vi "Scale sensor data.vi"(7 "Channel type":T1=enum."Flow meter", 11 "RAW Value":dbl) -> (2 "Type name":string, 3 "Scaled value":dbl)   [LabVIEW 2015]
uses:
  Channel type.ctl
  <vilib>/ptbypt/NI_PtbyPt.lvlib
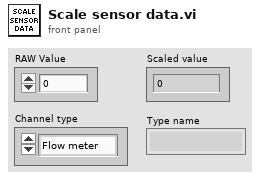
[diagram p1: front panel]
types:
  T1 = typedef "Channel type.ctl" = enum16{"Volts", "Flow meter", "Tank pressure", "Dewar level", "Raw ADC"}
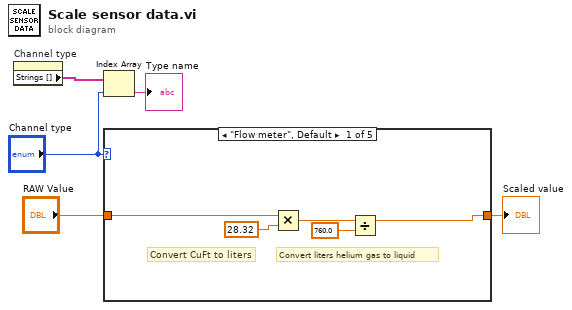
[diagram p0: block diagram]
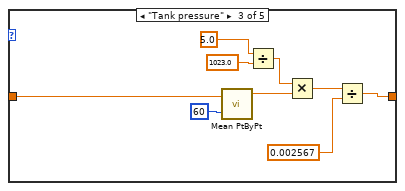
[diagram p3: hidden frame]
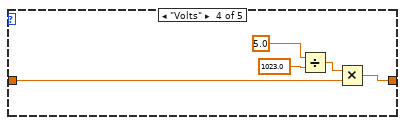
[diagram p4: hidden frame]
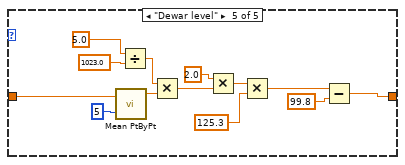
[diagram p5: hidden frame]
diagram:
  n1 = property on="Channel type" class="Enum (strict)"() -> ("Strings []"=w4:string[])  [unwired: 2 in, 2 out]
  n2 = Index Array(array=w4, index="Channel type") -> (element=→"Type name":string)
  n3 = case shown="\"Flow meter\", Default" "Channel type" {
    tunnel: [w7 w11 w12 w21 w26] -> w5
    tunnel: "RAW Value" -> [w9 w11 w18 w22 w37]
    frame "Flow meter", Default {
      # "Convert liters helium gas to liquid"
      # "Convert CuFt to liters"
      n4 = Multiply(x=w9, y=28.32) -> (x*y=w8:dbl)
      n5 = Divide(x=w8, y=760.0) -> (x/y=w7:dbl)
    }
    frame "Raw ADC" {
    }
    frame "Tank pressure" {
      n6 = call <vilib>:"Mean PtByPt.vi"("x"=w18, "sample length"=60) -> ("mean"=w19:dbl)  [unwired: 2 in, 1 out]
      n7 = Divide(x=5.0, y=1023.0) -> (x/y=w15:dbl)
      n8 = Multiply(x=w15, y=w19) -> (x*y=w13:dbl)
      n9 = Divide(x=w13, y=0.002567) -> (x/y=w12:dbl)
    }
    frame "Volts" {
      n10 = Divide(x=5.0, y=1023.0) -> (x/y=w23:dbl)
      n11 = Multiply(x=w23, y=w22) -> (x*y=w21:dbl)
    }
    frame "Dewar level" {
      n12 = call <vilib>:"Mean PtByPt.vi"("x"=w37, "sample length"=5) -> ("mean"=w34:dbl)  [unwired: 2 in, 1 out]
      n13 = Divide(x=5.0, y=1023.0) -> (x/y=w33:dbl)
      n14 = Multiply(x=w33, y=w34) -> (x*y=w27:dbl)
      n15 = Multiply(x=2.0, y=w27) -> (x*y=w29:dbl)
      n16 = Multiply(x=w29, y=125.3) -> (x*y=w31:dbl)
      n17 = Subtract(x=w31, y=99.8) -> (x-y=w26:dbl)
    }
  }
  "Scaled value" <- w5
